vi "Ridders Zero Finder (VI).vi"(6 "data":variant, 8 "f(x)":T1, 9 "end":dbl=1.0 format="%.2f", 10 "start":dbl format="%.2f", 11 "accuracy":dbl=1e-08 format="%.2e") -> (0 "error":i32, 1 "ticks":u32, 2 "f(zero)":dbl format="%.2f", 3 "zero":dbl format="%.2f")   [LabVIEW 2017, in "NI_Gmath.lvlib"]
doc: "Determines a zero of a 1D function in a given interval. The function has to be continuous and has to have different signs at the end points of the interval. You must manually select the polymorphic instance to use."
uses:
  <vilib>/gmath/NI_Gmath.lvlib
  <vilib>/gmath/_ref_NR.llb/functionRefnum.ctl
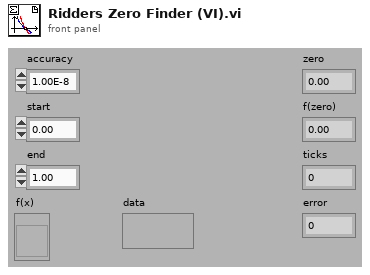
[diagram p1: front panel]
types:
  T1 = typedef "NI_Gmath.lvlib/functionRefnum.ctl" = refnum<vi>
  T2 = cluster{"f(x)":dbl, "f(x)":dbl, "start":dbl, "end":dbl}
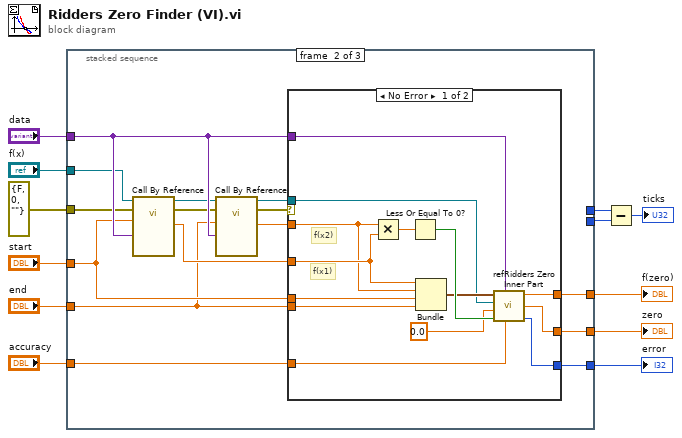
[diagram p0: block diagram]
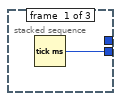
[diagram p2: hidden frame]
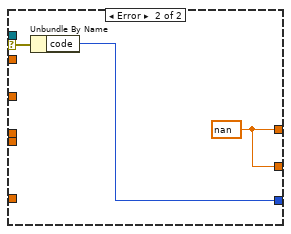
[diagram p3: hidden frame]
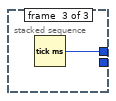
[diagram p4: hidden frame]
diagram:
  n1 = stacked-sequence {
    tunnel: "f(x)" -> [_ w26 _]
    tunnel: [_ w25 _] -> w12
    tunnel: [_ w24 _] -> w11
    tunnel: [_ w23 _] -> w10
    tunnel: errorcluster {"status"=FALSE, "code"=0, "source"=""} ("error out") -> [_ w22 _]
    tunnel: "start" -> [_ w21 _]
    tunnel: "data" -> [_ w28 _]
    tunnel: "end" -> [_ w19 _]
    tunnel: [w13 _ _] -> w3
    tunnel: [_ _ w46] -> w4
    tunnel: "accuracy" -> [_ w15 _]
    frame #0 {
      n2 = Tick Count (ms)() -> (millisecond timer value=w13:u32)
    }
    frame #1 {
      n3 = call-by-ref "?"(reference=w26, error in=w22, "Variant"=w28, "x"=w21) -> (reference out=w20:T1, error out=w17:errorcluster, 2:"f(x)"=w27:dbl)  [unwired: 3 in]
      n4 = call-by-ref "?"(reference=w20, error in=w17, "Variant"=w28, "x"=w19) -> (reference out=w14:T1, error out=w16:errorcluster, 2:"f(x)"=w18:dbl)  [unwired: 3 in]
      n5 = case shown="No Error" w16 {
        selector: w16 -> [_ w44]
        tunnel: w21 -> [w40 _]
        tunnel: w27 -> [w38 _]
        tunnel: [w34 w45] -> w25
        tunnel: [w33 w45] -> w24
        tunnel: [w32 w43] -> w23
        tunnel: w28 -> [w36 _]
        tunnel: w19 -> [w39 _]
        tunnel: w18 -> [w37 _]
        tunnel: w15 -> [w31 _]
        tunnel: w14 -> [w29 _]
        frame No Error {
          # "f(x1)"
          # "f(x2)"
          n6 = Multiply(x=w37, y=w38) -> (x*y=w41:dbl)
          n7 = Less Or Equal To 0?(x=w41) -> (x <= 0?=w42:bool)
          n8 = Bundle("f(x)"=w38, "f(x)"=w37, "start"=w40, "end"=w39) -> (w35:T2)  [unwired: 1 out]
          n9 = call <vilib>:"refRidders Zero Inner Part.vi"("start/end/f(x)"=w35, "Variant"=w36, "function refnum"=w29, "level"=0.0, "accuracy"=w31, "case"=w42) -> ("y value"=w34:dbl, "end"=w33:dbl, "error"=w32:i32)
        }
        frame Error {
          w45 = nan
          n10 = Unbundle By Name(w44) -> ("code"=w43:i32)
        }
      }
    }
    frame #2 {
      n11 = Tick Count (ms)() -> (millisecond timer value=w46:u32)
    }
  }
  "zero" <- w11
  "f(zero)" <- w12
  "error" <- w10
  n12 = Subtract(x=w4, y=w3) -> (x-y=→"ticks":u32)
